vi "FTW-CodeGen-Initialize.vi"(5 "XRef":refnum<vi>) -> (4 "State Out":T1)   [LabVIEW 2015, in "FTW-SQLite-Insert.xnode"]
uses:
  FTW-SQLite-Insert.xnode
  FTW-CodeGen-State.ctl
  FTW-CodeGen-XNodeCommonState.ctl
  FTW-CodeGen-Prototype.vi
panel:
  # "Inputs"
  # "Outputs"
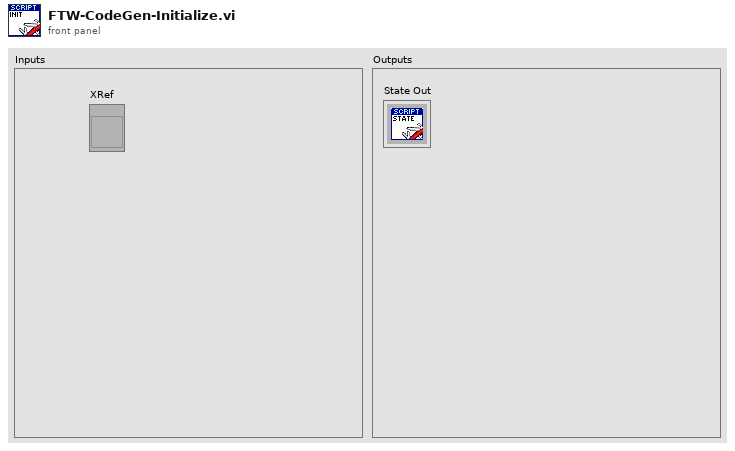
[diagram p1: front panel]
types:
  T1 = typedef "FTW-SQLite-Insert.xnode/FTW-CodeGen-State.ctl" = cluster{"Cache":T2}
  T2 = typedef "FTW-CodeGen-XNodeCommonState.ctl" = cluster{"Terms":cluster{"Name":string, "Id":string, "Type":variant, "Bounds":cluster{"Left":i32, "Top":i32, "Right":i32, "Bottom":i32}, "Input?":bool, "Required?":bool, "Recommended?":bool, "Adaptive?":bool, "Hidden?":bool, "Direction":enum32{"Auto", "Up", "Down", "Left", "Right", "Center"}, "Break Wire?":bool, "English Name":string}[], "AdaptiveTerms":string[], "AdaptedTypes":variant[], "ForceCodeRegeneration?":bool, "LastGeneration":timestamp, "Errors":string[]}
  T3 = cluster{"Name":string, "Id":string, "Type":variant, "Bounds":cluster{"Left":i32, "Top":i32, "Right":i32, "Bottom":i32}, "Input?":bool, "Required?":bool, "Recommended?":bool, "Adaptive?":bool, "Hidden?":bool, "Direction":enum32{"Auto", "Up", "Down", "Left", "Right", "Center"}, "Break Wire?":bool, "English Name":string}[]
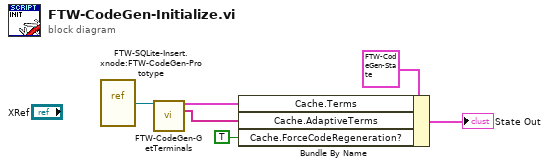
[diagram p0: block diagram]
diagram:
  n1 = vi-ref "FTW-SQLite-Insert.xnode:FTW-CodeGen-Prototype.vi"() -> (w6:refnum<vi>)
  n2 = call "FTW-CodeGen-GetTerminals.vi"("PrototypeVI"=w6) -> ("Terms"=w5:T3, "Adaptive Terminals"=w4:string[])  [unwired: 12 in, 1 out]
  n3 = Bundle By Name(cluster=T1 {"Cache"={"Terms"=[], "AdaptiveTerms"=[], "AdaptedTypes"=[], "ForceCodeRegeneration?"=FALSE, "LastGeneration"=timestamp(0 s since 1904-01-01), "Errors"=[]}} ("State Out"), "Cache.Terms"=w5, "Cache.AdaptiveTerms"=w4, "Cache.ForceCodeRegeneration?"=TRUE) -> (→"State Out":T1)
